vi "Send DBL Value.vi"(6 "Name (use label text)":string, 8 "error in (no error)":errorcluster, 9 "Value":dbl, 10 "DBL Refnum":refnum<vi>, 11 "Message Enqueuer in":refnum<class "Message Enqueuer.lvclass">) -> (0 "error out":errorcluster)   [LabVIEW 2015, in "ActorAutoRegistration.lvlib" / "DBLValueMsg.lvclass"]
uses:
  DBLValueMsg.lvclass
  <vilib>/ActorFramework/Message Enqueuer/Message Enqueuer.lvclass
  DBLValueMsg.lvclass/DBLValueMsg.ctl
  EventDataMessage/EventDataMessage.lvclass
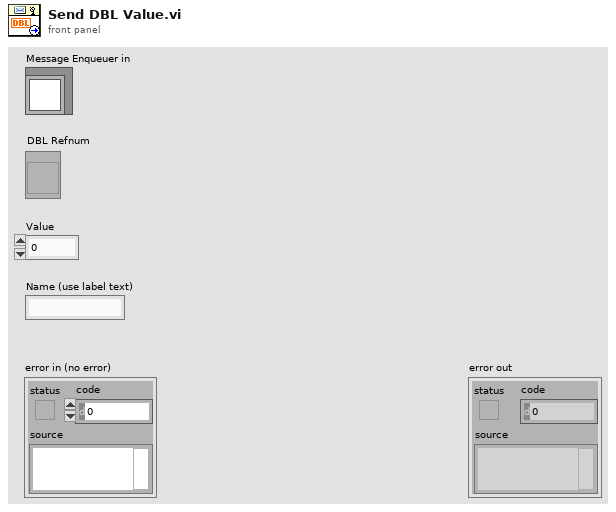
[diagram p1: front panel]
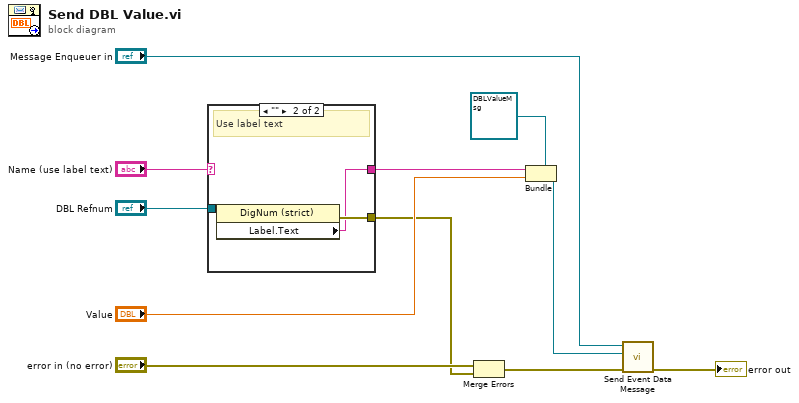
[diagram p0: block diagram]
diagram:
  n1 = case shown="\"\"" "Name (use label text)" {
    selector: "Name (use label text)" -> [w12 _]
    tunnel: [w12 w13] -> w11
    tunnel: "DBL Refnum" -> [_ w15]
    tunnel: [_ w14] -> w4
    frame Default {
      # "Use string provided"
    }
    frame "" {
      # "Use label text"
      n2 = property class="DigNum (strict)"(reference=w15) -> (error out=w14:errorcluster, "Label.Text"=w13:string)  [unwired: 1 in, 1 out]
    }
  }
  n3 = Merge Errors("error in (no error)", w4) -> (w5:errorcluster)
  n4 = Bundle(cluster=refnum<class "DBLValueMsg.lvclass"> refnum ("DBLValueMsg"), w11, "Value") -> (w2:refnum<class "DBLValueMsg.lvclass">)
  n5 = call "Send Event Data Message.vi"("error in (no error)"=w5, "EventDataMessage in"=w2, "Message Enqueuer in"="Message Enqueuer in") -> ("error out"=→"error out":errorcluster)  [unwired: 8 in]
